vi "LQR.vi"() -> ()   [LabVIEW 2019]
uses:
  <vilib>/Platform/TimedLoop/XDataNode/timing_clust.ctl
  <vilib>/Platform/TimedLoop/XDataNode/nitl_modes.ctl
  <vilib>/Platform/TimedLoop/XDataNode/wakeup.ctl
  <vilib>/Simulation/Shared/_Datatypes/SIM SISO Transfer Function.ctl
  <vilib>/myRIO/Instrument Drivers/Onboard IO/AI/typedefs/AI Reference.ctl
  <vilib>/myRIO/Common/Instrument Driver Framework/Utilities/typedefs/myRIO Generic Hardware Reference.ctl
  <vilib>/myRIO/Common/Instrument Driver Framework/Utilities/typedefs/Hardware Version Enum.ctl
  <vilib>/myRIO/Common/Instrument Driver Framework/Utilities/typedefs/myRIO v1.0 Reference.ctl
  <vilib>/myRIO/Common/Instrument Driver Framework/Utilities/typedefs/Generic FPGA Reference.ctl
  <vilib>/myRIO/Common/Instrument Driver Framework/myRIO v1.0/AI/typedefs/AI Channels List.ctl
  <vilib>/myRIO/Common/Instrument Driver Framework/myRIO v1.0/AI/typedefs/AI Channels Enum.ctl
  <vilib>/myRIO/Common/Instrument Driver Framework/Utilities/typedefs/Analog Scaling Constants List.ctl
  <vilib>/myRIO/Common/Instrument Driver Framework/Utilities/typedefs/Analog Scaling Constants.ctl
  <vilib>/userDefined/High Color/nirio_resource_hc.ctl
  <vilib>/myRIO/Instrument Drivers/Onboard IO/AO/typedefs/AO Reference.ctl
  <vilib>/myRIO/Common/Instrument Driver Framework/myRIO v1.0/AO/typedefs/AO Channels List.ctl
  <vilib>/myRIO/Common/Instrument Driver Framework/myRIO v1.0/AO/typedefs/AO Channels Enum.ctl
  <vilib>/myRIO/Common/Instrument Driver Framework/Utilities/vis/Is FPGA Ref Available.vi
  <vilib>/myRIO/Common/Instrument Driver Framework/myRIO v1.0/AI/vis/myRIO v1.1 Open AI.vi
  <vilib>/myRIO/Instrument Drivers/Onboard IO/AI/vis/Read.vi
  <vilib>/Simulation/DiscreteLinear/Implementation/NILVSim Discrete Transfer Function Direct.llb/SIM Discrete Transfer Function Diagram (SISO).vi
  <vilib>/myRIO/Common/Instrument Driver Framework/myRIO v1.0/AO/vis/myRIO v1.1 Open AO.vi
  <vilib>/myRIO/Instrument Drivers/Onboard IO/AO/vis/Write.vi
  <vilib>/myRIO/Common/Instrument Driver Framework/Utilities/vis/Validate Channels.vi
  <vilib>/myRIO/Common/Instrument Driver Framework/myRIO v1.0/AI/vis/myRIO v1.0 Reserve AI.vi
  <vilib>/Simulation/ContinuousLinear/Implementation/Shared/SIM Transfer Function Support.llb/SIM TransferFunction Normalize to Buffer.vi
  <vilib>/Simulation/DiscreteLinear/Implementation/Shared/SIM Init Discrete States.vi
  <vilib>/Simulation/DiscreteLinear/Implementation/NILVSim Discrete Transfer Function Direct.llb/SIM Transfer Function Direct core (SISO).vi
  <vilib>/myRIO/Common/Instrument Driver Framework/myRIO v1.0/AO/vis/myRIO v1.0 Reserve AO.vi
  <vilib>/myRIO/Common/Instrument Driver Framework/myRIO v1.0/AI/vis/myRIO v1.0 Build MUX Configuration AI.vi
  <vilib>/myRIO/Common/Instrument Driver Framework/myRIO v1.0/Resource Manager/vis/myRIO v1.0 Reserve Channel List.vi
  <vilib>/Simulation/ContinuousLinear/Implementation/Shared/SIM Transfer Function Support.llb/SIM TransferFunction Normalize.vi
  <vilib>/myRIO/Common/Instrument Driver Framework/myRIO v1.0/AO/vis/myRIO v1.0 Build MUX Configuration AO.vi
  <vilib>/myRIO/Common/Instrument Driver Framework/myRIO v1.0/Resource Manager/vis/myRIO v1.0 Reserve Channel.vi
  <vilib>/myRIO/Common/Instrument Driver Framework/myRIO v1.0/Resource Manager/vis/myRIO v1.0 Unreserve Channel.vi
  <vilib>/Simulation/Implementation/Shared/SIM Polynomials.llb/SIM Remove Zero Coefficients (DBL).vi
  <vilib>/myRIO/Common/Instrument Driver Framework/myRIO v1.0/Resource Manager/vis/myRIO v1.0 Build Mutex Name.vi
  <vilib>/Simulation/Implementation/Shared/SIM Polynomials.llb/SIM Divide Polynomials (DBL).vi
  <vilib>/Simulation/Implementation/Shared/SIM BuildSimErr.vi
  <vilib>/Utility/VariantDataType/GetNumericInfo.vi
  <vilib>/Utility/error.llb/Error Cluster From Error Code.vi
  <vilib>/myRIO/Common/Instrument Driver Framework/myRIO v1.0/myRIO v1.1 Open.vi
  <vilib>/myRIO/Common/Instrument Driver Framework/myRIO v1.0/AI/vis/myRIO v1.0 Get Scaling Constants AI.vi
  <vilib>/myRIO/Common/Instrument Driver Framework/Utilities/vis/IO Manager.vi
  <vilib>/myRIO/Common/Instrument Driver Framework/Utilities/vis/Configuration Manager.vi
  <vilib>/myRIO/Common/Instrument Driver Framework/myRIO v1.0/myRIO v1.0 Close.vi
  <vilib>/myRIO/Common/Instrument Driver Framework/myRIO v1.0/AI/vis/myRIO v1.0 Read AI.vi
  <vilib>/myRIO/Common/Instrument Driver Framework/myRIO v1.0/AO/vis/myRIO v1.0 Get Scaling Constants AO.vi
  <vilib>/myRIO/Common/Instrument Driver Framework/myRIO v1.0/AO/vis/myRIO v1.0 Write AO.vi
  <vilib>/platform/TimedLoop/XDataNode/XDataNode.xnode
  <vilib>/Simulation/Implementation/XNodeFramework/SimXNode/SimX.xnode
  <vilib>/myRIO/Express VI/Onboard IO/AI/AI Express VI.xnode
  <vilib>/myRIO/Instrument Drivers/Onboard IO/AI/vis/myRIO AI Open.xnode
  <vilib>/myRIO/Express VI/Onboard IO/AO/AO Express VI.xnode
  <vilib>/myRIO/Instrument Drivers/Onboard IO/AO/vis/myRIO AO Open.xnode
  <vilib>/Platform/TimedLoop/XDataNode/XDNodeRunTimeDep.lvlib
  <vilib>/myRIO/Instrument Drivers/Onboard IO/AI/AI.lvlib
  <vilib>/myRIO/Instrument Drivers/Onboard IO/AO/AO.lvlib
  <vilib>/ptbypt/NI_PtbyPt.lvlib
panel:
  out "Current Output EM 3":dbl(graph)=0.03990822535355048
  out "Current Output EM 2":dbl(graph)=0.03990822535355048
  in  "amplitude":dbl=1.0 format="%0.2f"
  out "Impulse Pattern":dbl(graph)
  in  "D":dbl=7.3
  in  "P":dbl=5291.0
  in  "stopNoise":bool=TRUE
  in  "gain_noise":dbl=0.2
  out "uniform white noise":dbl(graph)=-0.031193239239623867
  in  "AmpWhitehNoise":dbl=1.0 format="%0.2f"
  out "Iteration Duration":i64(graph)=347
  in  "Max FRF current 0-1000mA":dbl=4.0
  in  "Stop FRF":bool=TRUE
  in  "esc":bool
  out "scope":cluster{dbl, dbl, dbl, dbl, dbl}(graph)={-8.303163599999976, 0.03990822535355048, -0.0, -8.32082689025263, 946.4168275057085}
  out "Current Output EM":dbl(graph)=0.03990822535355048
  in  "Stop EM + FRF":bool=TRUE
  out "left[V]":dbl=-0.0
  out "right[V]":dbl=-0.0
  out "um":dbl=376.9531636
  # "mA"
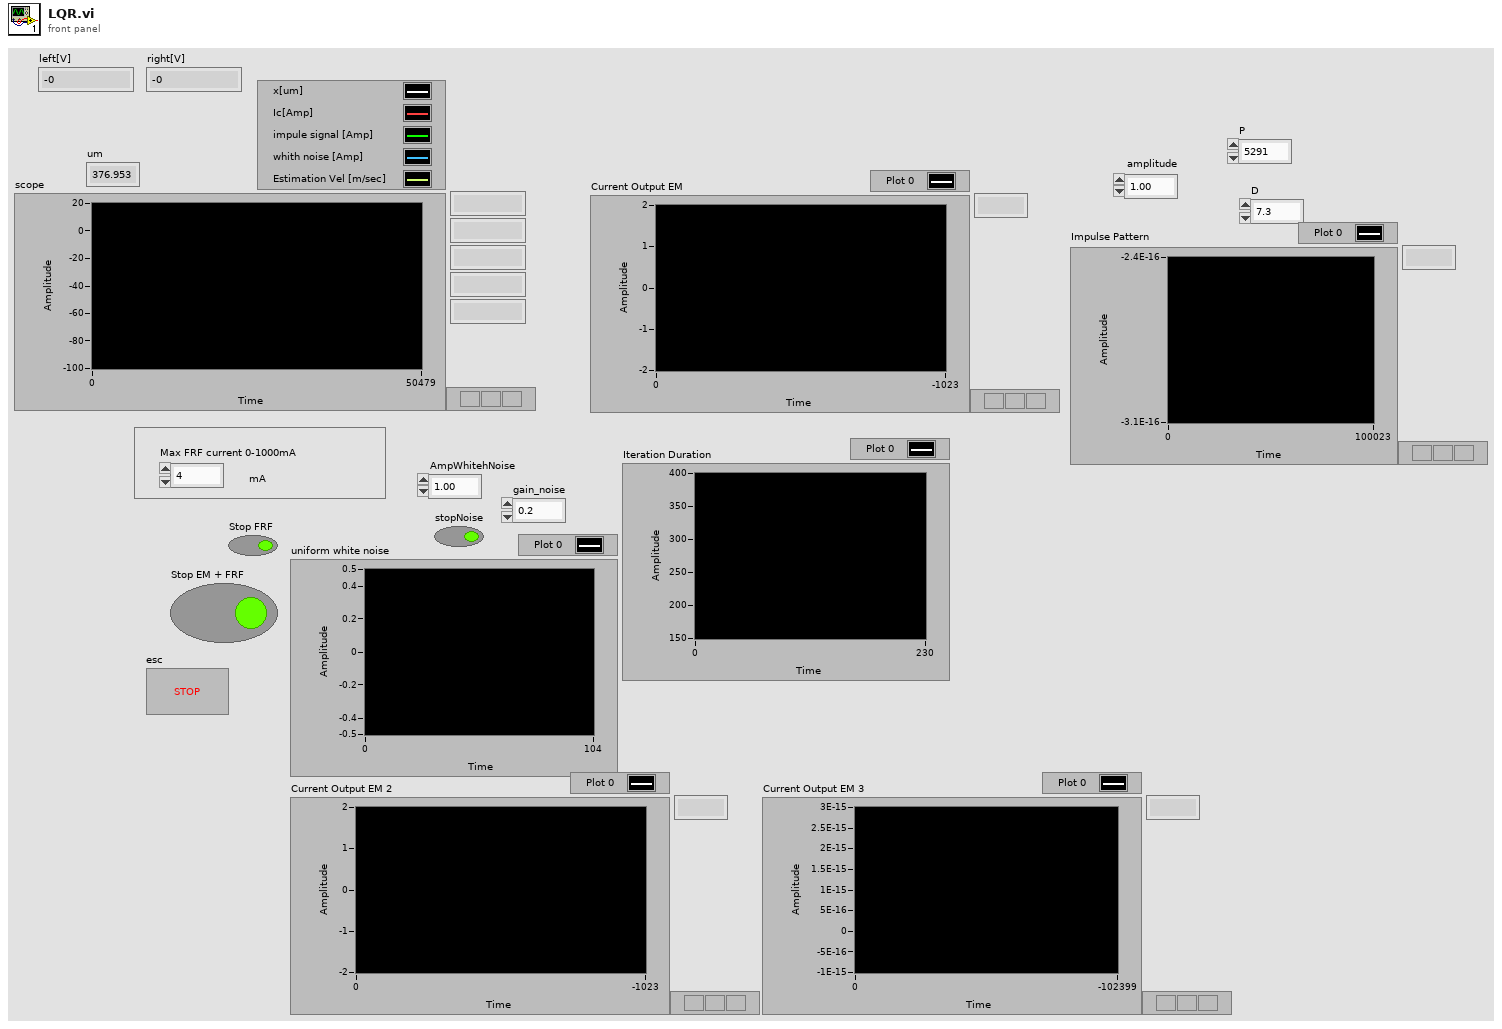
[diagram p1: front panel]
types:
  T1 = typedef "XDNodeRunTimeDep.lvlib/timing_clust.ctl" = cluster{"Expected End [f-1]":u64, "Actual End [f-1]":u64, "Finished Late? [f-1]":bool, "Expected End [i-1]":u64, "Actual End [i-1]":u64, "Finished Late? [i-1]":bool, "Expected Start [i]":u64, "Actual Start [i]":u64, "Expected Start [f]":u64, "Actual Start [f]":u64, "Source Name":string, "Structure Name":string, "Period":i64, "Deadline":i64, "Offset":i64, "Start":i64, "Priority":i32, "Timeout":i32, "Mode":T2, "Wakeup Reason":T3, "Error":errorcluster, "Source Type":string, "Secondary Source Type":string, "Global End Time":u64, "Global Start Time":u64, "Frame Duration":u64, "Iteration Duration":u64, "Assigned CPU":i32, "I/O Scan Engine Mode":u32}
  T2 = typedef "XDNodeRunTimeDep.lvlib/nitl_modes.ctl" = enum32{"No Change", "Process missed periods, maintain original phase", "Discard missed periods, maintain original phase", "Process missed periods, ignore original phase", "Discard missed periods, ignore original phase"}
  T3 = typedef "XDNodeRunTimeDep.lvlib/wakeup.ctl" = enum32{"Normal", "Aborted", "Asynchronous wakeup", "Timing source error", "Timed loop error", "Timeout"}
  T4 = typedef "SIM SISO Transfer Function.ctl" = cluster{"Numerator":dbl[], "Denominator":dbl[]}
  T5 = typedef "AI.lvlib/AI Reference.ctl" = cluster{"myRIO Reference":T6, "AI Channels List":T10, "AI Scaling Constants List":T12}
  T6 = typedef "myRIO Generic Hardware Reference.ctl" = cluster{"myRIO Model":T7, "myRIO Hardware Reference":T8}
  T7 = typedef "Hardware Version Enum.ctl" = enum16{"Unknown", "myRIO-1900", "myRIO-1950", "roboRIO", "NI ELVIS RIO CM", "ELVIS III"}
  T8 = typedef "myRIO v1.0 Reference.ctl" = cluster{"Generic FPGA Reference":T9, "Allow multiple opens":bool}
  T9 = typedef "Generic FPGA Reference.ctl" = refnum<k20>
  T10 = typedef "AI Channels List.ctl" = T11[]
  T11 = typedef "AI Channels Enum.ctl" = enum16{"Not Connected", "AudioIn/Left", "AudioIn/Right", "C/AI0", "C/AI1", "A/AI0", "A/AI1", "A/AI2", "A/AI3", "A/AI4", "A/AI5", "A/AI6", "A/AI7", "B/AI0", "B/AI1", "B/AI2", "B/AI3", "B/AI4", "B/AI5", "B/AI6", "B/AI7", "AI/AI0", "AI/AI1", "AI/AI2", "AI/AI3", "A/AI0 (DIFF)", "A/AI1 (DIFF)", "A/AI2 (DIFF)", "A/AI3 (DIFF)", "B/AI0 (DIFF)", "B/AI1 (DIFF)", "B/AI2 (DIFF)", "B/AI3 (DIFF)"}
  T12 = typedef "Analog Scaling Constants List.ctl" = T13[]
  T13 = typedef "Analog Scaling Constants.ctl" = cluster{"LSB Weight (Volts)":dbl, "Offset (Volts)":dbl, "Signed?":bool}
  T14 = typedef "nirio_resource_hc.ctl" = tag
  T15 = typedef "AO.lvlib/AO Reference.ctl" = cluster{"myRIO Reference":T6, "AO Channel List":T16, "AO Scaling Constant List":T12}
  T16 = typedef "AO Channels List.ctl" = T17[]
  T17 = typedef "AO Channels Enum.ctl" = enum16{"Not Connected", "AudioOut/Left", "AudioOut/Right", "C/AO0", "C/AO1", "A/AO0", "A/AO1", "B/AO0", "B/AO1"}
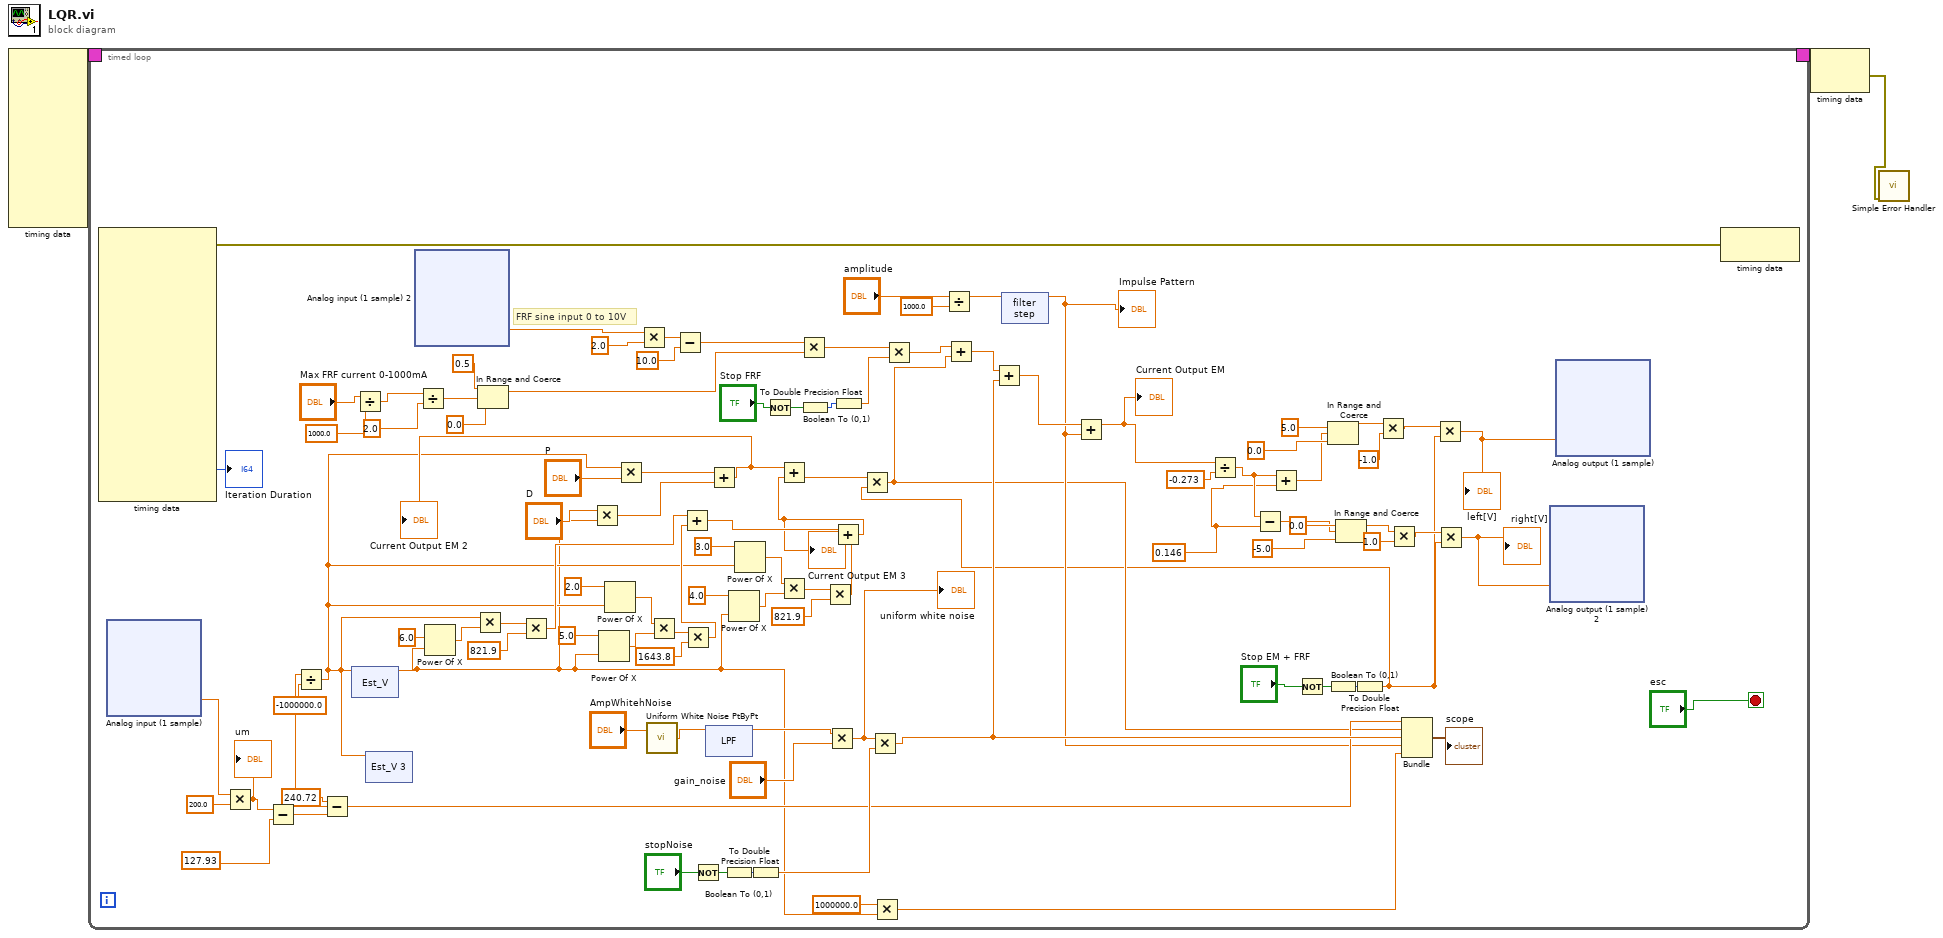
[diagram p0: block diagram]
diagram:
  n1 = node-c288() -> (w3:T1)  [unwired: 10 in]
  n2 = timed-loop {
    timing: w3 -> [_]
    timing-out: [_] -> w2
    stop <- "esc" stop-if-true
    w63 = 0.146 ("y")
    # "FRF sine input 0 to 10V"
    n3 = node-c288() -> (w104:errorcluster, →"Iteration Duration":i64)  [unwired: 1 in, 15 out]
    n4 = xnode "Analog input (1 sample)"() -> ("C/AI1 (AI1)"=w60:dbl)  [unwired: 1 in, 1 out]
    n5 = Multiply(x=w60, y=200.0) -> (x*y=w102:dbl)
    "um" <- w102
    n6 = Subtract(x=w102, y=127.93) -> (x-y=w101:dbl)
    n7 = Subtract(x=240.72, y=w101) -> (x-y=w43:dbl)
    n8 = Divide(x=w43, y=-1000000.0) -> (x/y=w5:dbl)
    n9 = xnode "Est_V"("input u(k)"=w5) -> ("output y(k)"=w4:dbl)  [unwired: 2 in, 1 out]
    n10 = Divide(x="Max FRF current 0-1000mA", y=1000.0) -> (x/y=w70:dbl)
    n11 = xnode "Est_V 3"("input u(k)"=w5) -> ()  [unwired: 2 in, 2 out]
    n12 = xnode "Analog input (1 sample) 2"() -> ("C/AI0 (AI0)"=w81:dbl)  [unwired: 1 in, 1 out]
    n13 = Divide(x=w70, y=2.0) -> (x/y=w74:dbl)
    n14 = Power Of X(1:w4, 2:6.0 ("y")) -> (0:w27:dbl)
    n15 = Multiply(x=w5, y=w27) -> (x*y=w26:dbl)
    n16 = In Range and Coerce(upper limit=0.5, x=w74, lower limit=0.0) -> (coerced(x)=w71:dbl)  [unwired: 1 out]
    n17 = Multiply(x=w26, y=821.9) -> (x*y=w12:dbl)
    n18 = Multiply(x="D", y=w4) -> (x*y=w41:dbl)
    n19 = Power Of X(1:w4, 2:5.0 ("y")) -> (0:w23:dbl)
    n20 = Power Of X(1:w5, 2:2.0 ("y")) -> (0:w19:dbl)
    n21 = Multiply(x=w5, y="P") -> (x*y=w42:dbl)
    n22 = Multiply(x=w81, y=2.0) -> (x*y=w79:dbl)
    n23 = call <vilib>:"Uniform White Noise PtByPt.vi"("amplitude"="AmpWhitehNoise") -> ("uniform white noise"=w53:dbl)  [unwired: 2 in]
    n24 = Multiply(x=w19, y=w23) -> (x*y=w22:dbl)
    n25 = Subtract(x=w79, y=10.0) -> (x-y=w76:dbl)
    n26 = Multiply(x=w22, y=1643.8) -> (x*y=w11:dbl)
    n27 = Add(x=w12, y=w11) -> (x+y=w10:dbl)
    n28 = Not(x="stopNoise") -> (.not. x?=w51:bool)
    n29 = xnode "LPF"("input u(k)"=w53) -> ("output y(k)"=w50:dbl)  [unwired: 2 in, 1 out]
    n30 = Add(x=w42, y=w41) -> (x+y=w7:dbl)
    "Current Output EM 2" <- w7
    n31 = Boolean To (0,1)(Boolean=w51) -> (0, 1=w52:i16)
    n32 = Power Of X(1:w4, 2:4.0 ("y")) -> (0:w17:dbl)
    n33 = Power Of X(1:w5, 2:3.0 ("y")) -> (0:w13:dbl)
    n34 = To Double Precision Float(number=w52) -> (double precision float=w47:dbl)
    n35 = Not(x="Stop FRF") -> (.not. x?=w84:bool)
    n36 = Multiply(x=w13, y=w17) -> (x*y=w16:dbl)
    n37 = Multiply(x=w76, y=w71) -> (x*y=w77:dbl)
    n38 = Boolean To (0,1)(Boolean=w84) -> (0, 1=w83:i16)
    n39 = Multiply(x=w16, y=821.9) -> (x*y=w9:dbl)
    n40 = Multiply(x=w50, y="gain_noise") -> (x*y=w46:dbl)
    "uniform white noise" <- w46
    n41 = Add(x=w10, y=w9) -> (x+y=w6:dbl)
    "Current Output EM 3" <- w6
    n42 = Add(x=w7, y=w6) -> (x+y=w8:dbl)
    n43 = To Double Precision Float(number=w83) -> (double precision float=w82:dbl)
    n44 = Multiply(x=w46, y=w47) -> (x*y=w45:dbl)
    n45 = Multiply(x=1000000.0, y=w4) -> (x*y=w32:dbl)
    n46 = Multiply(x=w77, y=w82) -> (x*y=w86:dbl)
    n47 = Divide(x="amplitude", y=1000.0) -> (x/y=w36:dbl)
    n48 = xnode "filter step"("input u(k)"=w36) -> ("output y(k)"=w33:dbl)  [unwired: 2 in, 1 out]
    "Impulse Pattern" <- w33
    n49 = Not(x="Stop EM + FRF") -> (.not. x?=w89:bool)
    n50 = Boolean To (0,1)(Boolean=w89) -> (0, 1=w91:i16)
    n51 = To Double Precision Float(number=w91) -> (double precision float=w29:dbl)
    n52 = Multiply(x=w8, y=w29) -> (x*y=w30:dbl)
    n53 = Add(x=w86, y=w30) -> (x+y=w44:dbl)
    n54 = Add(x=w44, y=w45) -> (x+y=w38:dbl)
    n55 = Add(x=w38, y=w33) -> (x+y=w34:dbl)
    "Current Output EM" <- w34
    n56 = Divide(x=w34, y=-0.273) -> (x/y=w64:dbl)
    n57 = Subtract(x=w64, y=w63) -> (x-y=w65:dbl)
    n58 = Add(x=w64, y=w63) -> (x+y=w66:dbl)
    n59 = In Range and Coerce(upper limit=5.0 ("x"), x=w66, lower limit=0.0) -> (coerced(x)=w57:dbl)  [unwired: 1 out]
    n60 = In Range and Coerce(upper limit=0.0 ("x"), x=w65, lower limit=-5.0) -> (coerced(x)=w94:dbl)  [unwired: 1 out]
    n61 = Multiply(x=w57, y=-1.0) -> (x*y=w62:dbl)
    n62 = Multiply(x=w94, y=1.0) -> (x*y=w61:dbl)
    n63 = Bundle(w43, w30, w45, "output y(k)"=w33, w32) -> (→"scope":cluster{dbl, dbl, dbl, "output y(k)":dbl, dbl})  [unwired: 1 in]
    n64 = Multiply(x=w62, y=w29) -> (x*y=w59:dbl)
    "left[V]" <- w59
    n65 = Multiply(x=w61, y=w29) -> (x*y=w58:dbl)
    "right[V]" <- w58
    n66 = xnode "Analog output (1 sample) 2"("C/AO1 (AO1)"=w58) -> ()  [unwired: 1 in, 1 out]
    n67 = xnode "Analog output (1 sample)"("C/AO0 (AO0)"=w59) -> ()  [unwired: 1 in, 1 out]
    n68 = node-c288(w104) -> ()  [unwired: 1 out]
  }
  n69 = node-c288(w2) -> (w1:errorcluster)
  n70 = call <vilib>:"Simple Error Handler.vi"("error in (no error)"=w1) -> ()  [unwired: 4 in, 5 out]
